vi "niScope Get Wfm Coefficients (poly).vi"   [LabVIEW 2011]
doc: "Returns coefficients that can be used to scale or normalize binary waveform data."
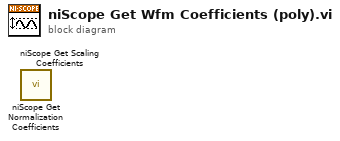
[diagram p0: block diagram]
diagram:
  n1 = call <instrlib>:"niScope Get Normalization Coefficients.vi"() -> ()  [unwired: 13 in, 3 out]
  n2 = call <instrlib>:"niScope Get Scaling Coefficients.vi"() -> ()  [unwired: 13 in, 3 out]
